vi "Destroy.vi"   [LabVIEW 2018, in "Toolkit.lvlib" / "Agent.lvclass"]
doc: "Deallocates, or frees, the memory allocated for the libssh2lv shared library Agent struct represented by this Agent object. After this is called, the object can no longer be used in the application without causing a segmentation fault, i.e. crashing LabVIEW. This VI must be called to avoid leaking memory or running Out-of-Memory (OOM) on resource-constrained systems."
uses:
  Agent.lvclass
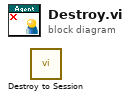
[diagram p0: block diagram]
diagram:
  n1 = call "Destroy to Session.vi"() -> ()  [unwired: 10 in, 2 out]
